vi "Variant to Class.vi"(8 "error in (no error)":errorcluster, 10 "Data in":variant, 11 "UTF Node in":refnum<class "UTF Node.lvclass">) -> (0 "error out":errorcluster, 2 "Data Out":variant, 3 "UTF Node out":refnum<class "UTF Node.lvclass">)   [LabVIEW 2014, in "UTF Node.lvclass"]
uses:
  UTF Node.lvclass
  Shared/Controls/Run UTF - STYP.ctl
  UTF Node.lvclass/UTF Node.ctl
  Classes/Build Job/Build Job.lvclass
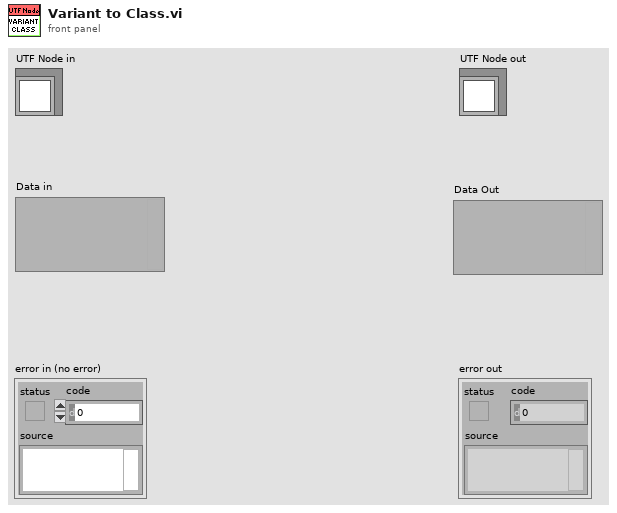
[diagram p1: front panel]
types:
  T1 = typedef "Run UTF - STYP.ctl" = cluster{"Project Path":string}
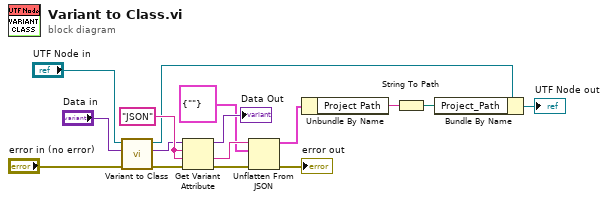
[diagram p0: block diagram]
diagram:
  w13 = "JSON" ("name")
  n1 = call-parent "Variant to Class.vi"("error in (no error)"="error in (no error)", "Data in"="Data in", "Build Job in"="UTF Node in") -> ("error out"=w12:errorcluster, "Data Out"=w11:variant, "Build Job out"=w3:refnum<class "UTF Node.lvclass">)  [unwired: 6 in]
  n2 = Get Variant Attribute(Variant=w11, name=w13, default value (empty Variant)=w13, error in=w12) -> (duplicate Variant=→"Data Out":variant, value=w8:string, error out=w9:errorcluster)  [unwired: 1 out]
  n3 = Unflatten From JSON(JSON string=w8, type and defaults=T1 {"Project Path"=""} ("Run UTF"), error in (no error)=w9) -> (value=w5:T1, error out=→"error out":errorcluster)  [unwired: 4 in]
  n4 = Unbundle By Name(w5) -> ("Project Path"=w4:string)
  n5 = String To Path(string=w4) -> (path=w2:path)
  n6 = Bundle By Name(cluster=w3, "Project_Path"=w2) -> (→"UTF Node out":refnum<class "UTF Node.lvclass">)
